vi "Ueberwachung_Fuehlerbruch.vi"(8 "Angehängtes Array":errorcluster[](array[cluster]), 11 "AI - TC Eingang":sgl[](array[numeric])) -> (0 "Fühlerbruch":bool[](array[boolean]), 2 "Temperaturen":sgl[](array[numeric]))   [LabVIEW 2020, in "Verwaltung - cRIO.lvlib"]
uses:
  Verwaltung - cRIO.lvlib
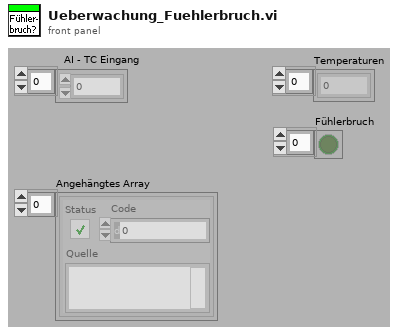
[diagram p1: front panel]
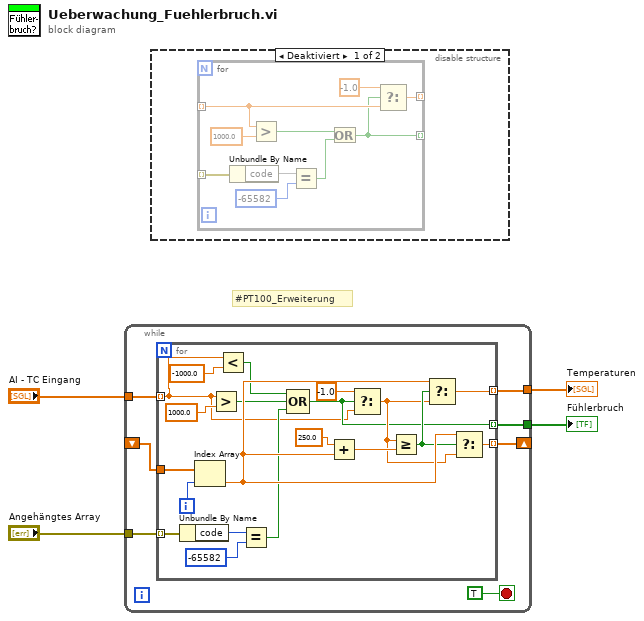
[diagram p0: block diagram]
diagram:
  # "#PT100_Erweiterung"
  n1 = while {
    tunnel: "AI - TC Eingang" -> [w10]
    tunnel: [w8] -> w4
    shift-right: [w9] -> _
    shift-left: _ -> [w7]
    tunnel: [w6] -> w3
    tunnel: "Angehängtes Array" -> [w5]
    stop <- TRUE stop-if-true
    n2 = for {
      tunnel: w10 -> [w13] mode=indexing
      tunnel: w7 -> [w31]
      tunnel: [w27] -> w8 mode=indexing
      tunnel: [w22] -> w9 mode=indexing
      tunnel: [w15] -> w6 mode=indexing
      tunnel: w5 -> [w18] mode=indexing
      i -> [w28]
      n3 = Unbundle By Name(w18) -> ("code"=w19:i32)
      n4 = Index Array(array=w31, index=w28) -> (element=w24:sgl)
      n5 = Greater?(x=w13, y=sgl 1000.0) -> (0:w17:bool)
      n6 = Less?(x=w13, y=sgl -1000.0) -> (x < y?=w12:bool)
      n7 = Equal?(x=w19, y=-65582) -> (x = y?=w16:bool)
      n8 = Compound Arithmetic op=OR ("Mehrfacharithmetik")(w12, w17, w16) -> (w15:bool)
      n9 = Add(x=sgl 250.0 ("y"), y=w24) -> (x+y=w25:sgl)
      n10 = Select(t=sgl -1.0, s=w15, f=w13) -> (s? t:f=w21:sgl)
      n11 = Greater Or Equal?(x=w21, y=w25) -> (x >= y?=w23:bool)
      n12 = Select(t=w24, s=w23, f=w21) -> (s? t:f=w27:sgl)
      n13 = Select(t=w24, s=w23, f=w21) -> (s? t:f=w22:sgl)
    }
  }
  "Temperaturen" <- w4
  "Fühlerbruch" <- w3
  n14 = disable-structure shown="Deaktiviert" {
    frame Disabled {
      n15 = for {
        tunnel: [w39] -> _ mode=indexing
        tunnel: _ -> [w38] mode=indexing
        tunnel: [w32] -> _ mode=indexing
        tunnel: _ -> [w37] mode=indexing
        n16 = Unbundle By Name(w37) -> ("code"=w36)
        n17 = Greater?(x=w38, y=sgl 1000.0) -> (0:w34:bool)
        n18 = Equal?(x=w36, y=-65582) -> (x = y?=w33:bool)
        n19 = Or(x=w34, y=w33) -> (x .or. y?=w32:bool)
        n20 = Select(t=sgl -1.0, s=w32, f=w38) -> (s? t:f=w39:sgl)
      }
    }
    frame Enabled {
    }
  }
